vi "Create Agent Public Key Refnum.vi"(7 "agent":T1, 8 "error in (no error)":errorcluster, 11 "libssh2_agent_publickey*":u64 format="%.0x") -> (0 "error out":errorcluster, 3 "agent public key":T2)   [LabVIEW 2017, in "libssh2.lvlib"]
doc: "Creates a <B>public key</B> refnum from a pointer to libssh2_agent_publickey."
uses:
  libssh2.lvlib
  Agent Public Key Refnum.ctl
  Agent Refnum.ctl
  Agent Public Key Refnum Data.ctl
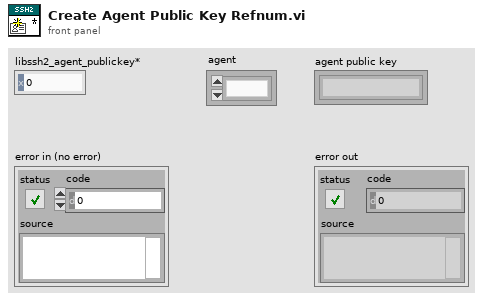
[diagram p1: front panel]
types:
  T1 = typedef "libssh2.lvlib/Agent Refnum.ctl" = refnum<k1>
  T2 = typedef "libssh2.lvlib/Agent Public Key Refnum.ctl" = refnum<k1>
  T3 = typedef "libssh2.lvlib/Agent Public Key Refnum Data.ctl" = cluster{"libssh2_agent_publickey*":u64, "agent":T1}
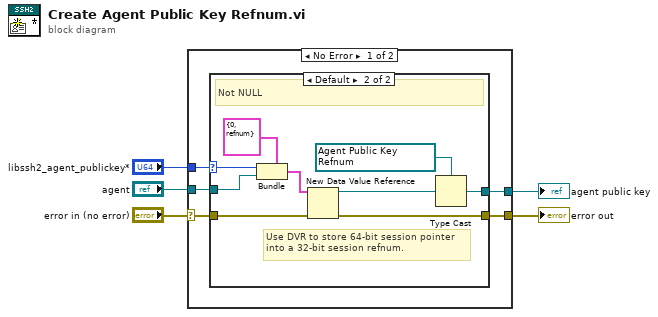
[diagram p0: block diagram]
diagram:
  n1 = case shown="No Error" "error in (no error)" {
    selector: "error in (no error)" -> [w8 w21]
    tunnel: [w10 _] -> w5
    tunnel: [w9 w21] -> w4
    tunnel: "libssh2_agent_publickey*" -> [w7 _]
    tunnel: "agent" -> [w6 _]
    frame No Error {
      n2 = case shown="Default" w7 {
        selector: w7 -> [_ w18]
        tunnel: [_ w19] -> w10
        tunnel: [w11 w16] -> w9
        tunnel: w8 -> [w11 w15]
        tunnel: w6 -> [_ w12]
        frame 0 {
          # "NULL"
        }
        frame Default {
          w20 = T2 refnum items=["agent publickey"] ("libssh2_agent_publickey_refnum")
          # "Use DVR to store 64-bit session pointer\ninto a 32-bit session refnum."
          # "Not NULL"
          n3 = Bundle(cluster=T3 {"libssh2_agent_publickey*"=0, "agent"=refnum} ("agent public key data"), "libssh2_agent_publickey*"=w18, "agent"=w12) -> (w14:T3)
          n4 = New Data Value Reference(data value=w14, error in=w15) -> (data value reference=w17:refnum<data-value>, error out=w16:errorcluster)
          n5 = Type Cast(type=w20, x=w17) -> (*(type *) &x=w19:T2)
        }
      }
    }
    frame Error {
    }
  }
  "agent public key" <- w5
  "error out" <- w4
